vi "clFile_writeStr.vi"(9 "offset (0)":u32, 10 "new substring":string, 11 "clFile.lvclass":refnum<class "clFile.lvclass">) -> (3 "clFile.lvclass 2":refnum<class "clFile.lvclass">)   [LabVIEW 2020, in "vi_lib.lvlib" / "clFile.lvclass"]
uses:
  clFile.lvclass
  clFile.lvclass/clFile.ctl
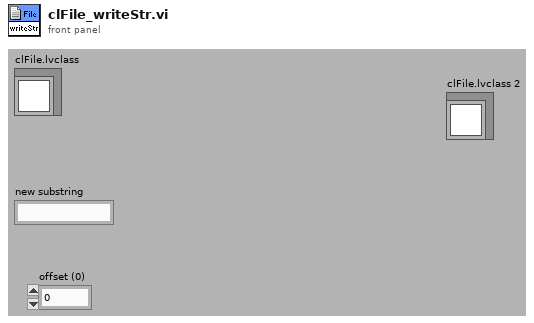
[diagram p1: front panel]
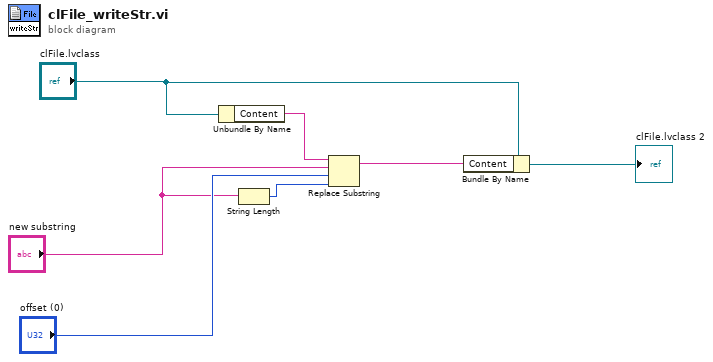
[diagram p0: block diagram]
diagram:
  n1 = Unbundle By Name("clFile.lvclass") -> ("Content"=w2:string)
  n2 = String Length(string="new substring") -> (length=w3:i32)
  n3 = Replace Substring(2:w3, 3:"offset (0)", 4:"new substring", 5:w2) -> (1:w1:string)  [unwired: 1 out]
  n4 = Bundle By Name(cluster="clFile.lvclass", "Content"=w1) -> (→"clFile.lvclass 2":refnum<class "clFile.lvclass">)
